vi "Surface_AxesScale.vi"(8 "Y-axis Max":dbl, 9 "X-axis max":dbl, 10 "3D Surface":refnum<k7>(container), 11 "Auto Scale":bool) -> ()   [LabVIEW 2018]
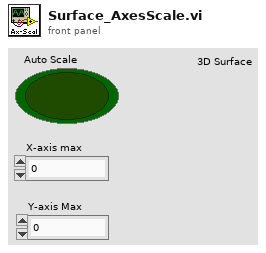
[diagram p1: front panel]
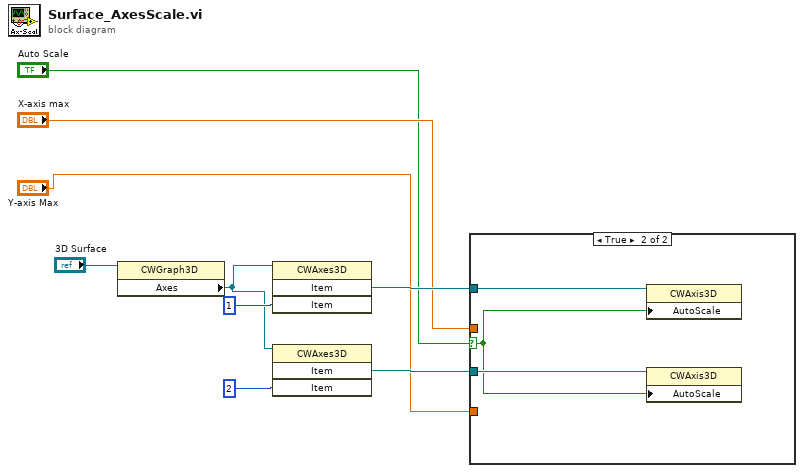
[diagram p0: block diagram]
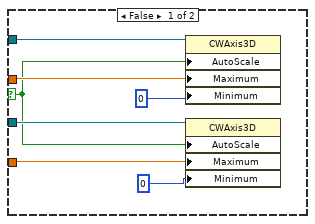
[diagram p2: hidden frame]
diagram:
  n1 = property class="CWGraph3D"(reference="3D Surface") -> ("Axes"=w5:refnum<k7>)  [unwired: 1 in, 2 out]
  n2 = invoke class="CWAxes3D" method="Item"(reference=w5, "Item"=1) -> ("Item"=w9:refnum<k7>)  [unwired: 2 in, 3 out]
  n3 = invoke class="CWAxes3D" method="Item"(reference=w5, "Item"=2) -> ("Item"=w6:refnum<k7>)  [unwired: 2 in, 3 out]
  n4 = case shown="True" "Auto Scale" {
    selector: "Auto Scale" -> [w12 w17]
    tunnel: w9 -> [w16 w19]
    tunnel: w6 -> [w15 w18]
    tunnel: "Y-axis Max" -> [w14 _]
    tunnel: "X-axis max" -> [w13 _]
    frame False {
      n5 = property class="CWAxis3D"(reference=w16, "AutoScale"=w12, "Maximum"=w13, "Minimum"=0) -> ()  [unwired: 1 in, 2 out]
      n6 = property class="CWAxis3D"(reference=w15, "AutoScale"=w12, "Maximum"=w14, "Minimum"=0) -> ()  [unwired: 1 in, 2 out]
    }
    frame True {
      n7 = property class="CWAxis3D"(reference=w19, "AutoScale"=w17) -> ()  [unwired: 1 in, 2 out]
      n8 = property class="CWAxis3D"(reference=w18, "AutoScale"=w17) -> ()  [unwired: 1 in, 2 out]
    }
  }
